vi "16.vi"() -> ()   [LabVIEW 2021]
panel:
  out "Sum of Digits":i32
  in  "N (for 2^N)":i32
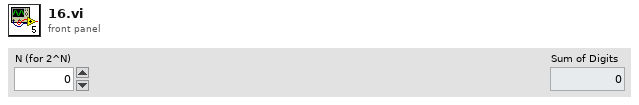
[diagram p1: front panel]
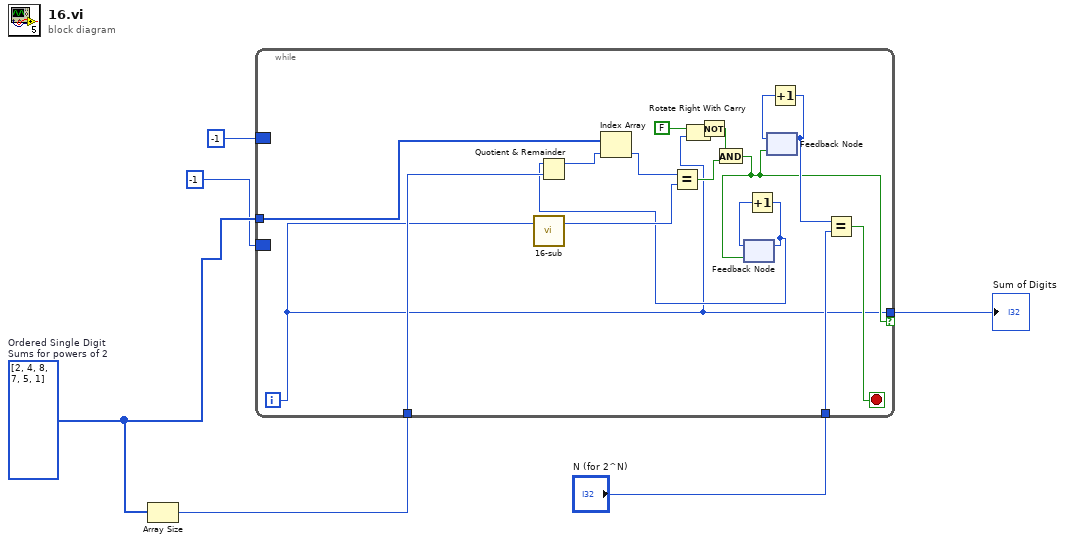
[diagram p0: block diagram]
diagram:
  w4 = u64[] [2, 4, 8, 7, 5, 1]  # Ordered Single Digit Sums for powers of 2
  n1 = Array Size(array=w4) -> (size(s)=w3:i32)
  n2 = while {
    tunnel: w4 -> [w19]
    tunnel: "N (for 2^N)" -> [w21]
    tunnel: [w7] -> w5 if=w8
    tunnel: w3 -> [w18]
    border: -1 -> [_]
    border: -1 -> [_]
    i -> [w7]
    stop <- w20 stop-if-true
    n3 = call "16-sub.vi"("Number"=w7) -> ("Single Digit Sum"=w16:u64)  [unwired: 2 in]
    n4 = Rotate Right With Carry(2:w7, 3:FALSE ("carry")) -> (1:w11:bool)  [unwired: 1 out]
    n5 = Not(x=w11) -> (.not. x?=w9:bool)
    n6 = feedback #1() -> (w15:i32)
    n7 = Increment(x=w15) -> (x+1=w14:i32)
    n8 = Quotient & Remainder(x=w14, y=w18) -> (x-y*floor(x/y)=w17:i32)  [unwired: 1 out]
    n9 = Index Array(array=w19, index=w17) -> (element=w13:u64)
    n10 = Equal?(x=w13, y=w16) -> (x = y?=w10:bool)
    n11 = And(x=w9, y=w10) -> (x .and. y?=w8:bool)
    n12 = feedback-in #1(w14, w8) -> ()
    n13 = feedback #2() -> (w23:i32)
    n14 = Increment(x=w23) -> (x+1=w22:i32)
    n15 = feedback-in #2(w22, w8) -> ()
    n16 = Equal?(x=w22, y=w21) -> (x = y?=w20:bool)
  }
  "Sum of Digits" <- w5
